vi "Data Access Through Reference.vi"(9 "Time Out In ms":i32=-1, 11 "DVR In":refnum<data-value>) -> (0 "Time Out":bool, 2 "Data Out":T1, 3 "DVR Out":refnum<data-value>)   [LabVIEW 2019, in "1D U16 Group With ID DVR Queue.lvclass"]
uses:
  1D U16 Group With ID DVR Queue.lvclass
  Type Def/Data Type.ctl
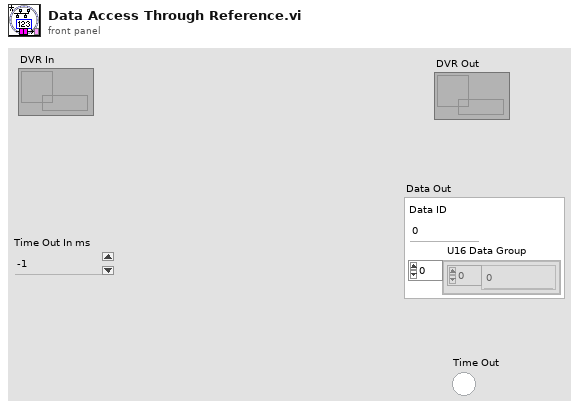
[diagram p1: front panel]
types:
  T1 = typedef "Data Type.ctl" = cluster{"Data ID":i64, "U16 Data Group":cluster{"Array":u16[]}[]}
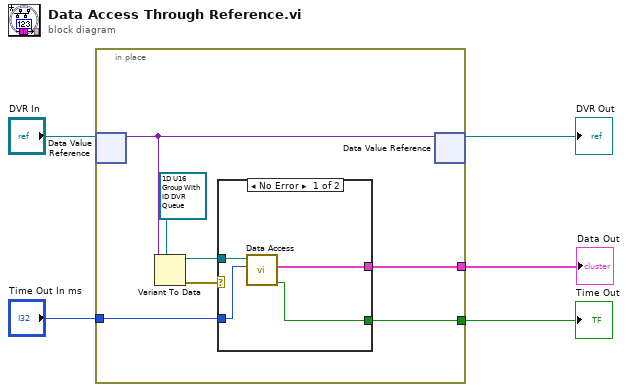
[diagram p0: block diagram]
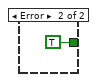
[diagram p2: hidden frame]
diagram:
  n1 = in-place {
    in-place-border: "Time Out In ms" -> [w9]
    in-place-border: [w8] -> w2
    in-place-border: [w6] -> w1
    n2 = in-place-dvr #1("DVR In") -> (w12:variant)  [unwired: 1 out]
    n3 = Variant To Data(type=refnum<class "1D U16 Group With ID DVR Queue.lvclass"> refnum ("1D U16 Group With ID DVR Queue.lvclass"), Variant=w12) -> (data=w10:refnum<class "1D U16 Group With ID DVR Queue.lvclass">, error out=w11:errorcluster)  [unwired: 1 in]
    n4 = case shown="No Error" w11 {
      tunnel: w10 -> [w16 _]
      tunnel: w9 -> [w15 _]
      tunnel: [w14 TRUE ("Time Out")] -> w8
      tunnel: [w13 _] -> w6
      frame No Error {
        n5 = call "Data Access.vi"("Time Out In ms"=w15, "1D U16 Group With ID DVR Queue in"=w16) -> ("Time Out"=w14:bool, "Data Out"=w13:T1)  [unwired: 7 in, 1 out]
      }
      frame Error {
      }
    }
    n6 = in-place-dvr #1(w12) -> (→"DVR Out":refnum<data-value>)  [unwired: 1 out]
  }
  "Time Out" <- w2
  "Data Out" <- w1
